vi "strain_to_playback_speed.vi"(11 "Waveform":waveform(dbl)) -> (3 "playback speed":dbl)   [LabVIEW 2022 SP3]
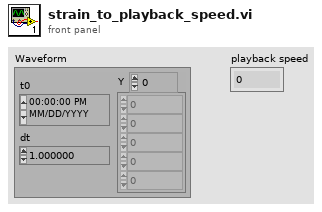
[diagram p1: front panel]
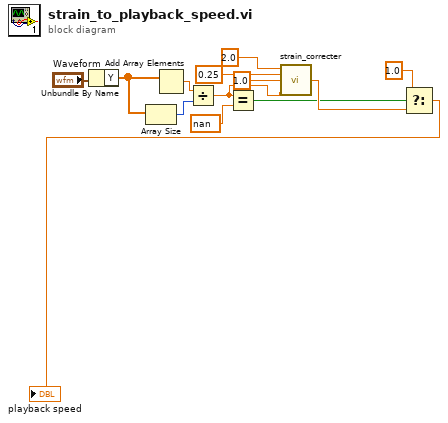
[diagram p0: block diagram]
diagram:
  n1 = Unbundle By Name("Waveform") -> ("Y"=w2:dbl[])
  n2 = Array Size(array=w2) -> (size(s)=w4:i32)
  n3 = Add Array Elements(numeric array=w2) -> (sum=w3:dbl)
  n4 = Divide(x=w3, y=w4) -> (x/y=w12:dbl)
  n5 = Equal?(x=w12, y=nan) -> (x = y?=w6:bool)
  n6 = call "strain_correcter.vi"("max"=2.0, "min"=0.25, "normal"=1.0, "Raw strain"=w12) -> ("strain"=w10:dbl)  [unwired: 11 in]
  n7 = Select(t=1.0, s=w6, f=w10) -> (s? t:f=→"playback speed":dbl)
